vi "ramp_el.vi"(6 "ramp tail (s)":dbl=5e-06 format="%#_6p", 8 "dt":dbl=5e-08 caption="dt (s)" format="%#_6p", 9 "ramp head (s)":dbl=5e-06 format="%#_6p", 10 "wf_in":dbl[][](array[numeric])) -> (0 "num_tail":i32, 1 "num_head":i32, 2 "wf_out":dbl[][](array[numeric]))   [LabVIEW 2013, in "wf_tools.lvlib"]
uses:
  wf_tools.lvlib
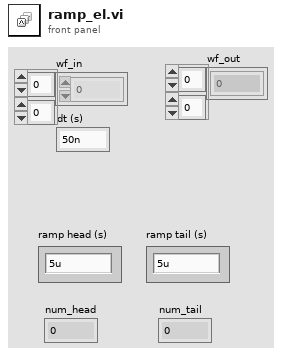
[diagram p1: front panel]
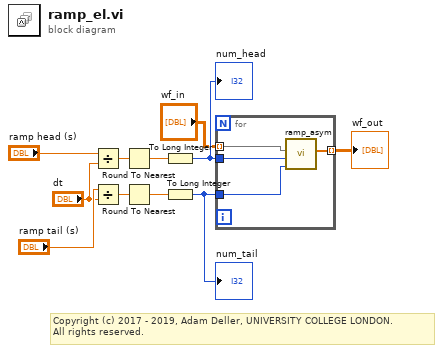
[diagram p0: block diagram]
diagram:
  # "Copyright (c) 2017 - 2019, Adam Deller, UNIVERSITY COLLEGE LONDON.\nAll rights reserved."
  n1 = Divide(x="ramp head (s)", y="dt") -> (x/y=w9:dbl)
  n2 = Divide(x="ramp tail (s)", y="dt") -> (x/y=w3:dbl)
  n3 = Round To Nearest(number=w9) -> (nearest integer value=w10:dbl)
  n4 = Round To Nearest(number=w3) -> (nearest integer value=w2:dbl)
  n5 = To Long Integer(number=w10) -> (32bit integer=w11:i32)
  "num_head" <- w11
  n6 = To Long Integer(number=w2) -> (32bit integer=w1:i32)
  "num_tail" <- w1
  n7 = for {
    tunnel: "wf_in" -> [w15] mode=indexing
    tunnel: [w14] -> w6 mode=indexing
    tunnel: w11 -> [w13]
    tunnel: w1 -> [w12]
    n8 = call "ramp_asym.vi"("num_tail"=w12, "num_head"=w13, "wf_in"=w15) -> ("wf_out"=w14:dbl[])  [unwired: 8 in]
  }
  "wf_out" <- w6
